vi "Delete existing tags.vi"(8 "error in (no error)":errorcluster, 11 "Item Ref in":T1 format="%.0x") -> (0 "error out":errorcluster, 3 "Item Ref out":T1 format="%.0x")   [LabVIEW 2023, in "Ethernet IP Custom Device Custom Device.lvlib"]
uses:
  Ethernet IP Custom Device Custom Device.lvlib
  <vilib>/NI VeriStand/Custom Device API/Custom Device Item Ref.ctl
  <vilib>/NI VeriStand/Custom Device Tools/Custom Device Utility Library/NI VeriStand - Search for Item by Name.vi
  <vilib>/NI VeriStand/Custom Device Tools/Custom Device Utility Library/Custom Device Utility Library.lvlib
  <vilib>/NI VeriStand/Custom Device API/Custom Device API.lvlib
panel:
  in  "sections (Inputs,Outputs)":string[](array[string])=["Inputs", "Outputs"]
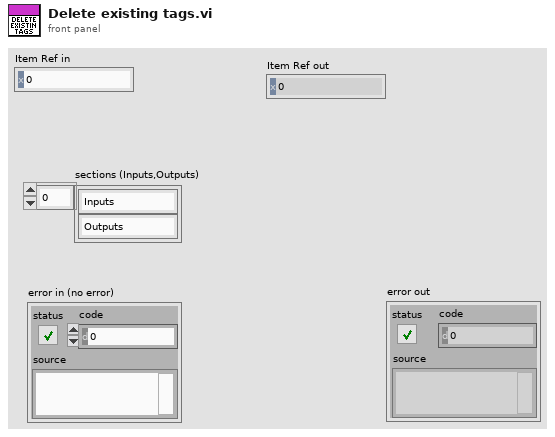
[diagram p1: front panel]
types:
  T1 = typedef "Custom Device API.lvlib/Custom Device Item Ref.ctl" = u64
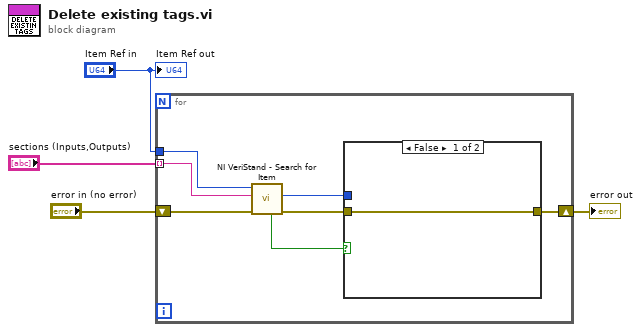
[diagram p0: block diagram]
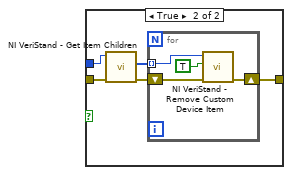
[diagram p2: hidden frame]
diagram:
  n1 = for {
    tunnel: "Item Ref in" -> [w11]
    tunnel: "sections (Inputs,Outputs)" -> [w9] mode=indexing
    shift-right: [w5] -> w2
    shift-left: "error in (no error)" -> [w10]
    n2 = call-poly <vilib>:"NI VeriStand - Search for Item.vi"("error in"=w10, "Item Name"=w9, "Section Ref in"=w11) -> ("error out"=w6:errorcluster, "Item Ref"=w7:T1, "Found"=w8:bool)  [unwired: 5 in, 1 out]
    n3 = case shown="False" w8 {
      tunnel: w7 -> [_ w16]
      tunnel: w6 -> [w12 w17]
      tunnel: [w12 w13] -> w5
      frame False {
      }
      frame True {
        n4 = call <vilib>:"NI VeriStand - Get Item Children.vi"("error in (no error)"=w17, "Item Ref in"=w16) -> ("error out"=w15:errorcluster, "Child Refs"=w14:T1[])  [unwired: 6 in, 2 out]
        n5 = for {
          shift-right: [w18] -> w13
          shift-left: w15 -> [w20]
          tunnel: w14 -> [w19] mode=indexing
          n6 = call <vilib>:"NI VeriStand - Remove Custom Device Item.vi"("error in (no error)"=w20, "Force Delete (F)"=TRUE, "Item Ref in"=w19) -> ("error out"=w18:errorcluster)  [unwired: 7 in, 1 out]
        }
      }
    }
  }
  "error out" <- w2
  "Item Ref out" <- "Item Ref in"
